vi "Stop Core.vi"(10 "final error code":i32, 11 "Task in":refnum<class "Task.lvclass">) -> (3 "Task out":refnum<class "Task.lvclass">)   [LabVIEW 2020, in "Volatus.lvlib" / "Task.lvclass"]
doc: "(<B>Filename</B>: Actor Framework.lvlib:Actor.lvclass:Stop Core.vi)\n\nDefines what the actor does before it stops. Use the <B>final error code</B> input to determine whether the actor shut down in response to an error.\n\nBy default, this method passes the Stop message along to all auto-stop nested actors. A descendant class may override this method to define additional behavior, such as shutting down any processes the actor initiated in its override of the Actor Core method."
uses:
  Task.lvclass
  C:/Program Files (x86)/National Instruments/LabVIEW 2020/vi.lib/ActorFramework/Actor/Actor.lvclass
  Task State.ctl
  API/API.lvclass
  <vilib>/ActorFramework/Actor/Actor.lvclass/Actor.ctl
  Task.lvclass/Task.ctl
  APIRegistrationHandler Messages/Unregister API Msg/Unregister API Msg.lvclass/Unregister API Msg.ctl
  <vilib>/ActorFramework/Message Enqueuer/Message Enqueuer.lvclass/Message Enqueuer.ctl
  <vilib>/ActorFramework/Message Enqueuer/Enqueue.vi
  APIRegistrationHandler Messages/Unregister API Msg/Unregister API Msg.lvclass
  C:/Program Files (x86)/National Instruments/LabVIEW 2020/vi.lib/ActorFramework/Message/Message.lvclass
  <vilib>/ActorFramework/Message Priority Queue/Priority Enqueue.vi
  <vilib>/ActorFramework/Actor/Actor.lvclass
  Volatus.lvlib
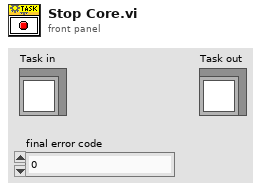
[diagram p1: front panel]
types:
  T1 = typedef "Volatus.lvlib/Task State.ctl" = enum16{"Unknown", "Idle", "Initializing", "Starting", "Running", "Stopping", "Stopped", "Error - Init", "Error - Start", "Error - Run", "Error - Stop"}
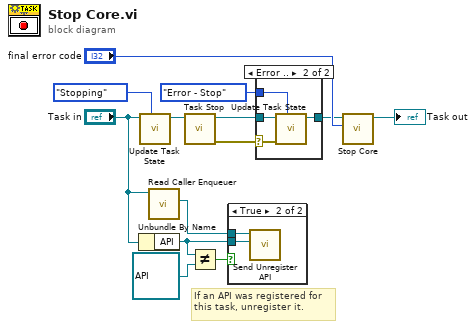
[diagram p0: block diagram]
diagram:
  # "If an API was registered for this task, unregister it."
  n1 = Unbundle By Name("Task in") -> ("API"=w2:refnum<class "API.lvclass">)
  n2 = call "Update Task State.vi"("State"=Task_State."Stopping", "Task in"="Task in") -> ("Task out"=w11:refnum<class "Task.lvclass">)  [unwired: 8 in, 1 out]
  n3 = call <vilib>:"Read Caller Enqueuer.vi"("Actor"="Task in") -> ("Caller Enqueuer"=w1:refnum<class "Message Enqueuer.lvclass">)  [unwired: 10 in]
  n4 = call "Task Stop.vi"("Task in"=w11) -> ("error out"=w9:errorcluster, "Task out"=w8:refnum<class "Task.lvclass">)  [unwired: 9 in]
  n5 = Not Equal?(x=w2, y=refnum<class "API.lvclass"> refnum) -> (x != y?=w3:bool)
  n6 = case shown="True" w3 {
    tunnel: w2 -> [_ w15]
    tunnel: w1 -> [_ w14]
    frame False {
    }
    frame True {
      n7 = call "Send Unregister API.vi"("API"=w15, "Message Enqueuer"=w14) -> ()  [unwired: 8 in, 2 out]
    }
  }
  n8 = case shown="Error .." w9 {
    selector: w9 -> [_ w19]
    tunnel: w8 -> [w16 w20]
    tunnel: [w16 w18] -> w6
    tunnel: Task_State."Error - Stop" ("State") -> [_ w17]
    frame No Error {
    }
    frame Error {
      n9 = call "Update Task State.vi"("State"=w17, "error in (no error)"=w19, "Task in"=w20) -> ("Task out"=w18:refnum<class "Task.lvclass">)  [unwired: 7 in, 1 out]
    }
  }
  n10 = call-parent "Stop Core.vi"("final error code"="final error code", "Actor in"=w6) -> ("Actor out"=→"Task out":refnum<class "Task.lvclass">)  [unwired: 9 in]
